vi "Example - Building a PPL.vi"() -> ()   [LabVIEW 2020]
doc: "Demonstrates the use of the Application Builder API to create and build a Packed Library build specification."
uses:
  <vilib>/AppBuilder/AB_API/common/AB_API Version Number.ctl
  <vilib>/AppBuilder/AB_API/PPL/NI_AB_API_PPL.lvclass
panel:
  out "Generated Files":path[](array[path])
  # "Overview: Demonstrates the use of the Application Builder API to create and build a Packed Library build specification.\nRequirements: LabVIEW Professional Development System or LabVIEW Application Builder\nInstructions:\n1. Run the VI. A Packed Library build specification will be created, which will then be built programmatically.\n2. Examine the PPL build specification in the new project.\n3. Close the temporary project and delete the temporary project files generated by this example when you are done."
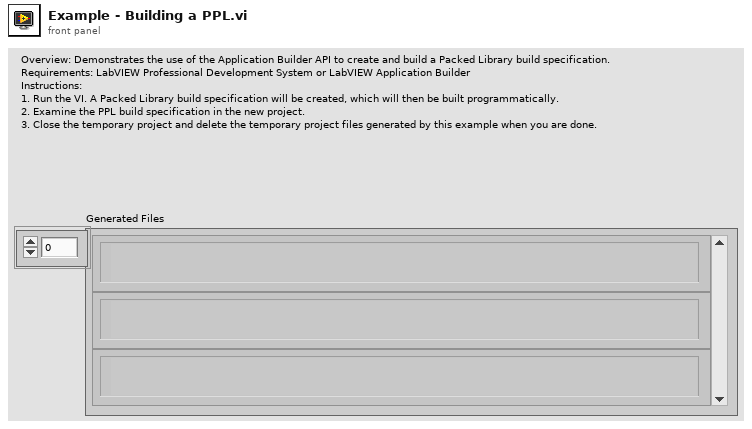
[diagram p1: front panel]
types:
  T1 = typedef "AB_API Version Number.ctl" = cluster{"Major":u16, "Minor":u16, "Fix":u16, "Build":u16}
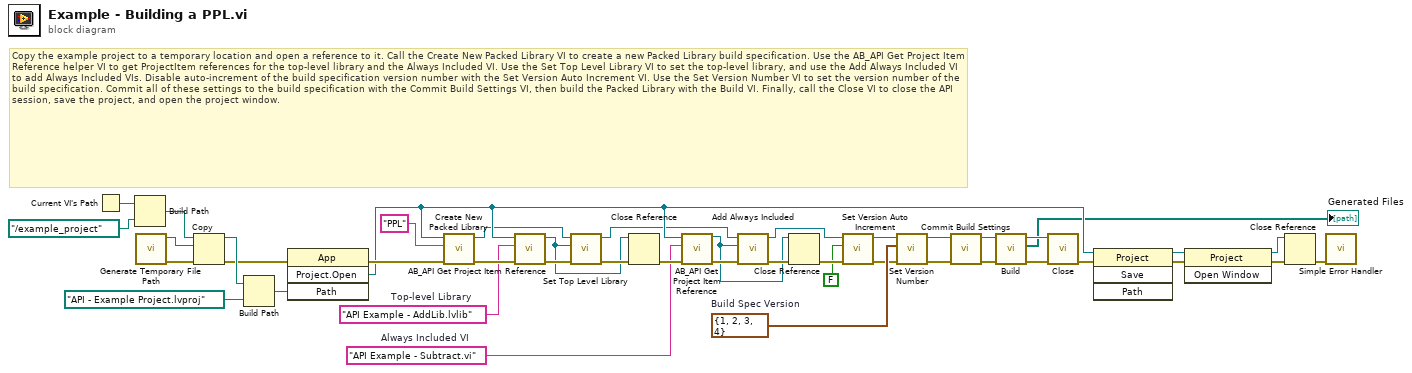
[diagram p0: block diagram]
diagram:
  w8 = T1 {"Major"=1, "Minor"=2, "Fix"=3, "Build"=4}  # Build Spec Version
  w13 = "API Example - Subtract.vi"  # Always Included VI
  w22 = "API Example - AddLib.lvlib"  # Top-level Library
  # "Copy the example project to a temporary location and open a reference to it. Call the Create New Packed Library VI to create a new Packed Library build specification. Use the AB_API Get Project Item Reference helper VI to get ProjectItem references for the top-level library and the Always Included VI. Use the Set Top Level Library VI to set the top-level library, and use the Add Always Included VI to add Always Included VIs. Disable auto-increment of the build specification version number with the Set Version Auto Increment VI. Use the Set Version Number VI to set the version number of the build specification. Commit all of these settings to the build specification with the Commit Build Settings VI, then build the Packed Library with the Build VI. Finally, call the Close VI to close the API session, save the project, and open the project window."
  n1 = Current VI's Path() -> (path=w42:path)
  n2 = Build Path(base path=w42, name or relative path=path "../example_project" ("path")) -> (appended path=w39:path)
  n3 = call <vilib>:"Generate Temporary File Path.vi"() -> ("error out"=w32:errorcluster, "Unique Temporary File Path"=w38:path)  [unwired: 10 in]
  n4 = Copy(8:w32, 10:w38, 11:w39) -> (0:w31:errorcluster, 3:w37:path)  [unwired: 2 in, 1 out]
  n5 = Build Path(base path=w37, name or relative path=path "API - Example Project.lvproj") -> (appended path=w35:path)
  n6 = invoke class="App" method="Project.Open"(error in=w31, "Path"=w35) -> (error out=w41:errorcluster, "Project:Open"=w34:refnum<vi>)  [unwired: 2 in, 2 out]
  n7 = call <vilib>:"Create New Packed Library.vi"("error in (no error)"=w41, "Build specification name"="PPL", "Project Refnum"=w34) -> ("error out"=w24:errorcluster, "PPL out"=w12:refnum<class "NI_AB_API_PPL.lvclass">)  [unwired: 7 in]
  n8 = call <vilib>:"AB_API Get Project Item Reference.vi"("error in (no error)"=w24, "Name"=w22, "Project Refnum"=w34) -> ("error out"=w21:errorcluster, "ProjectItem Refnum"=w19:refnum<vi>)  [unwired: 6 in, 1 out]
  n9 = call-dynamic "Set Top Level Library.vi"("error in (no error)"=w21, "ProjectItem Refnum"=w19, "PPL in"=w12) -> ("error out"=w20:errorcluster, "PPL out"=w11:refnum<class "NI_AB_API_PPL.lvclass">)  [unwired: 7 in]
  n10 = Close Reference(reference=w19, error in (no error)=w20) -> (error out=w18:errorcluster)
  n11 = call <vilib>:"AB_API Get Project Item Reference.vi"("error in (no error)"=w18, "Name"=w13, "Project Refnum"=w34) -> ("error out"=w16:errorcluster, "ProjectItem Refnum"=w14:refnum<vi>)  [unwired: 6 in, 1 out]
  n12 = call-dynamic "Add Always Included.vi"("error in (no error)"=w16, "ProjectItem Refnum"=w14, "PPL in"=w11) -> ("error out"=w15:errorcluster, "PPL out"=w6:refnum<class "NI_AB_API_PPL.lvclass">)  [unwired: 7 in]
  n13 = Close Reference(reference=w14, error in (no error)=w15) -> (error out=w17:errorcluster)
  n14 = call-dynamic "Set Version Auto Increment.vi"("error in (no error)"=w17, "Auto Increment Version"=FALSE, "NI_AB_API_PPL in"=w6) -> ("error out"=w7:errorcluster, "NI_AB_API_PPL out"=w5:refnum<class "NI_AB_API_PPL.lvclass">)  [unwired: 7 in]
  n15 = call-dynamic "Set Version Number.vi"("error in (no error)"=w7, "Version number"=w8, "PPL in"=w5) -> ("error out"=w10:errorcluster, "PPL out"=w9:refnum<class "NI_AB_API_PPL.lvclass">)  [unwired: 7 in]
  n16 = call-dynamic "Commit Build Settings.vi"("error in (no error)"=w10, "PPL in"=w9) -> ("error out"=w30:errorcluster, "PPL out"=w28:refnum<class "NI_AB_API_PPL.lvclass">)  [unwired: 8 in]
  n17 = call-dynamic "Build.vi"("error in (no error)"=w30, "PPL in"=w28) -> ("error out"=w29:errorcluster, "GeneratedFiles"=→"Generated Files":path[], "PPL out"=w27:refnum<class "NI_AB_API_PPL.lvclass">)  [unwired: 6 in, 1 out]
  n18 = call-dynamic "Close.vi"("error in (no error)"=w29, "DLL in"=w27) -> ("error out"=w26:errorcluster)  [unwired: 9 in]
  n19 = invoke class="Project" method="Save"(reference=w34, error in=w26) -> (reference out=w2:refnum<vi>, error out=w43:errorcluster)  [unwired: 2 in, 2 out]
  n20 = invoke class="Project" method="Open Window"(reference=w2, error in=w43) -> (reference out=w1:refnum<vi>, error out=w3:errorcluster)  [unwired: 1 in, 1 out]
  n21 = Close Reference(reference=w1, error in (no error)=w3) -> (error out=w40:errorcluster)
  n22 = call <vilib>:"Simple Error Handler.vi"("error in (no error)"=w40) -> ()  [unwired: 4 in, 5 out]
